vi "Setup.vi"(7 "Actor":refnum<class "Actor.lvclass">) -> (4 "Error":errorcluster, 5 "Actor":refnum<class "Actor.lvclass">)   [LabVIEW 2020, in "_Template.lvlib" / "{{Actor}}.lvlib" / "Actor.lvclass"]
uses:
  Actor.lvclass
  Actor.lvclass/Actor.ctl
  jettl/jettl/Actor/Actor.lvclass
panel:
  # "This front panel should not be manipulated."
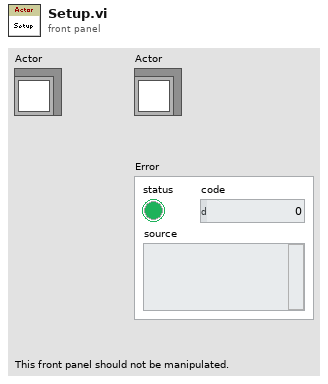
[diagram p1: front panel]
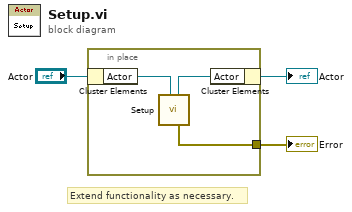
[diagram p0: block diagram]
diagram:
  # "Extend functionality as necessary."
  n1 = in-place {
    in-place-border: [w4] -> w1
    n2 = in-place-cluster #1("Actor") -> ("Actor"=w6:refnum<class "Actor.lvclass">)
    n3 = call-dynamic "Setup.vi"("Actor"=w6) -> ("Error"=w4:errorcluster, "Actor"=w5:refnum<class "Actor.lvclass">)  [unwired: 9 in]
    n4 = in-place-cluster #1("Actor"=w5) -> (→"Actor":refnum<class "Actor.lvclass">)
  }
  "Error" <- w1
